vi "uTTA_SetMode.vi"(4 "error in":errorcluster, 6 "OperatingMode":T1, 7 "VISA Refnum in":refnum<visa-resource-name>) -> (0 "error out":errorcluster, 2 "Received":string, 3 "VISA Refnum out":refnum<visa-resource-name>)   [LabVIEW 2021]
uses:
  uTTA_Controls/CTL_uTTA_OperatingMode.ctl
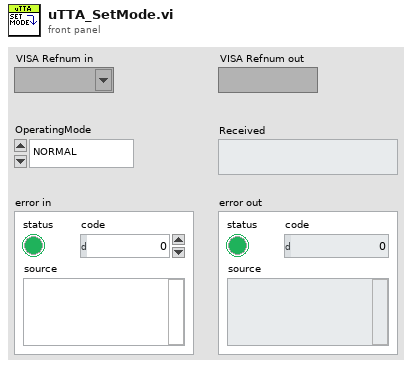
[diagram p1: front panel]
types:
  T1 = typedef "CTL_uTTA_OperatingMode.ctl" = enum16{"NORMAL", "TEST_MODE", "TEMP_CONTROL"}
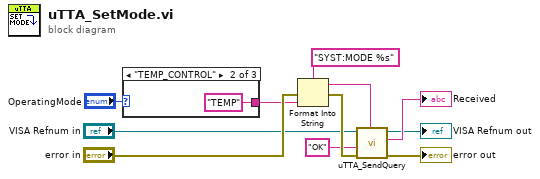
[diagram p0: block diagram]
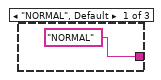
[diagram p2: hidden frame]
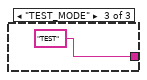
[diagram p3: hidden frame]
diagram:
  n1 = case shown="\"TEMP_CONTROL\"" "OperatingMode" {
    tunnel: ["NORMAL" ("input 1") "TEMP" ("input 1") "TEST" ("input 1")] -> w2
    frame "NORMAL", Default {
    }
    frame "TEMP_CONTROL" {
    }
    frame "TEST_MODE" {
    }
  }
  n2 = Format Into String(format string="SYST:MODE %s", error in="error in", w2) -> (resulting string=w8:string, error out=w10:errorcluster)  [unwired: 1 in]
  n3 = call "uTTA_SendQuery.vi"("Send String"=w8, "error in (no error)"=w10, "Response Qualifier(\"\")"="OK" ("Response Qualifier(\"\")"), "VISA Refnum in"="VISA Refnum in") -> ("error out"=→"error out":errorcluster, "Received"=→"Received":string, "VISA Refnum out"=→"VISA Refnum out":refnum<visa-resource-name>)  [unwired: 5 in]
